vi "Write configuration.vi"(8 "error in":errorcluster, 10 "configuration":refnum<class "NISE_CEF_serializable configuration.lvclass">, 11 "Device in":refnum<class "Device.lvclass">) -> (0 "error out":errorcluster, 3 "Device out":refnum<class "Device.lvclass">)   [LabVIEW 2014, in "Device.lvclass"]
uses:
  Device.lvclass
  <vilib>/NI/Configuration Framework/serializable configuration/NISE_CEF_serializable configuration.lvclass
  Device Configuration/Device Configuration.lvclass
  Device.lvclass/Device.ctl
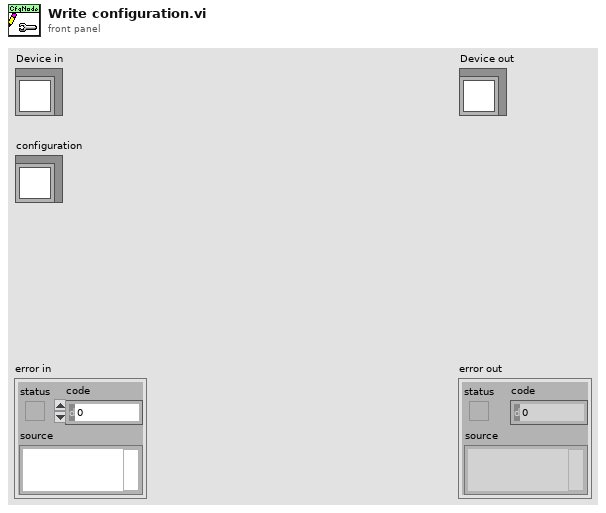
[diagram p1: front panel]
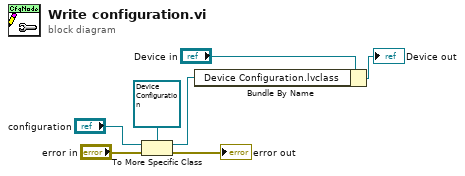
[diagram p0: block diagram]
diagram:
  n1 = To More Specific Class(target class=refnum<class "Device Configuration.lvclass"> refnum ("Device Configuration.lvclass"), reference="configuration", error in="error in") -> (specific class reference=w1:refnum<class "Device Configuration.lvclass">, error out=→"error out":errorcluster)
  n2 = Bundle By Name(cluster="Device in", "Device Configuration.lvclass"=w1) -> (→"Device out":refnum<class "Device.lvclass">)
